vi "Transcriptor LabVIEW to VHDL code Step 0 Create Definitions.vi"(8 "error in":errorcluster, 11 "Diagram in":refnum<vi>) -> (0 "error out":errorcluster, 3 "structure definition cluster":T1)   [LabVIEW 2018]
uses:
  types/LabVIEW Universal Transcriptor Structure Definitions.ctl
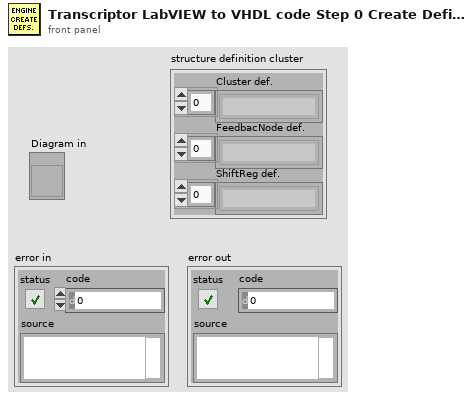
[diagram p1: front panel]
types:
  T1 = typedef "LabVIEW Universal Transcriptor Structure Definitions.ctl" = cluster{"Cluster def.":string[], "FeedbacNode def.":string[], "ShiftReg def.":string[]}
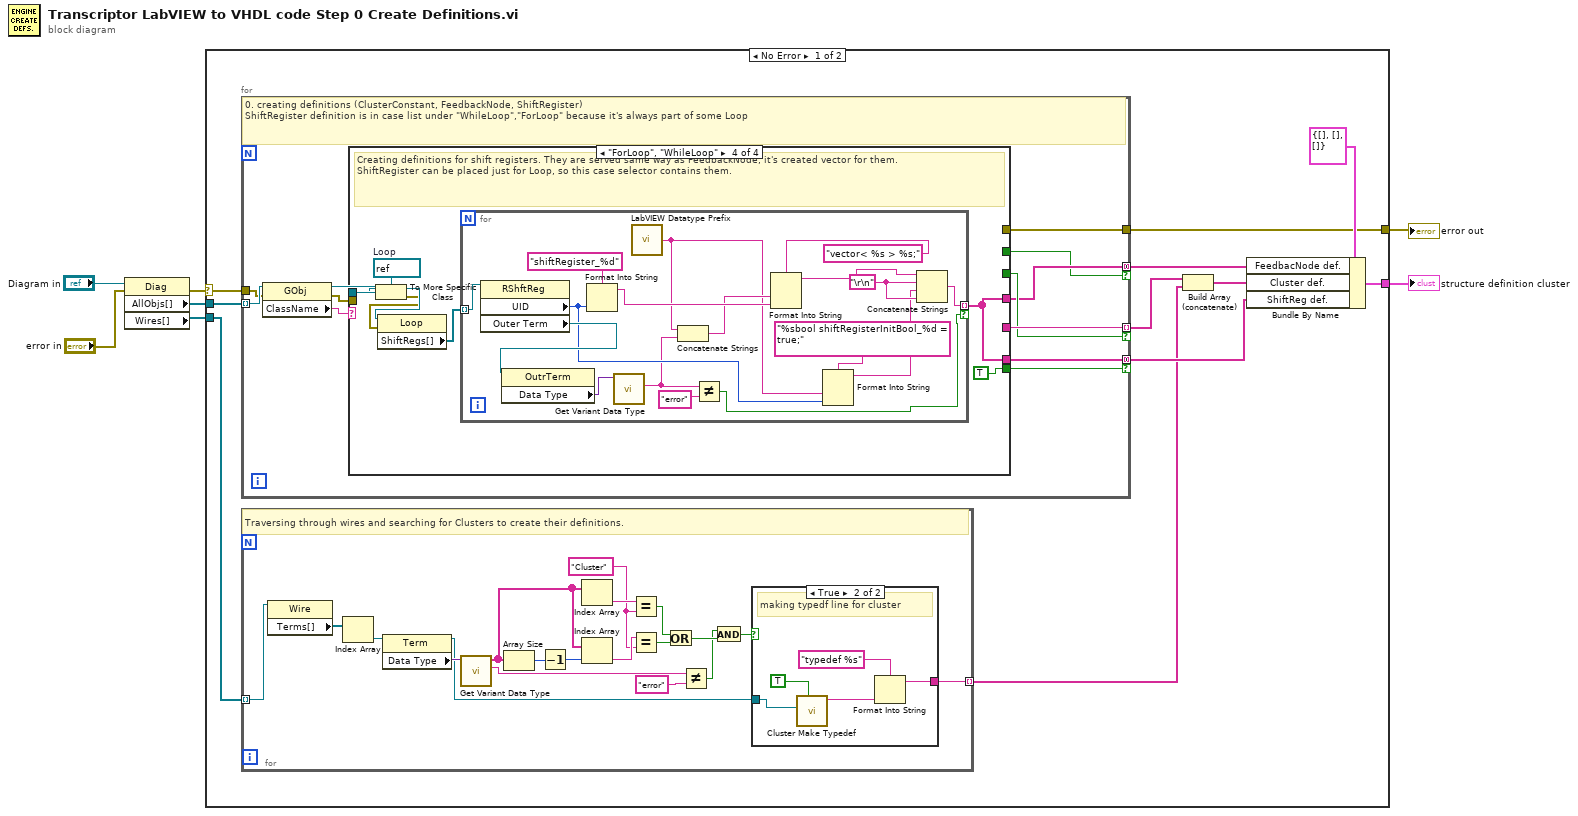
[diagram p0: block diagram]
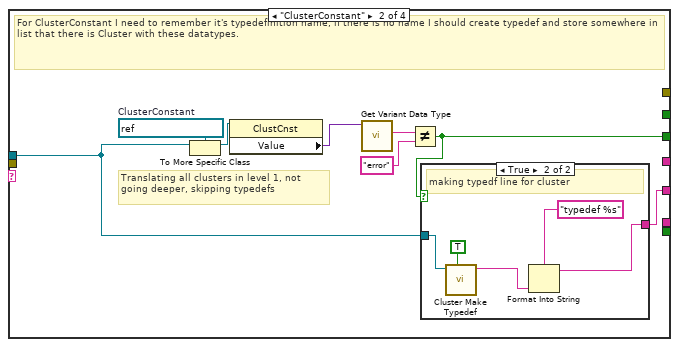
[diagram p4: hidden frame]
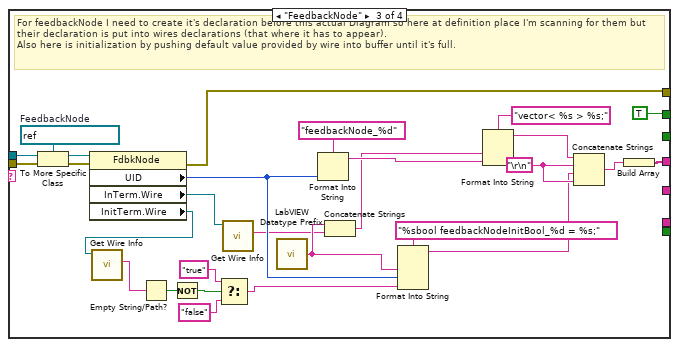
[diagram p6: hidden frame]
diagram:
  n1 = property class="Diag"(reference="Diagram in", error in="error in") -> (error out=w4:errorcluster, "AllObjs[]"=w7:refnum<vi>[], "Wires[]"=w1:refnum<vi>[])  [unwired: 1 out]
  n2 = case shown="No Error" w4 {
    selector: w4 -> [w14 w120]
    tunnel: [w18 _] -> w2
    tunnel: w7 -> [w15 _]
    tunnel: [w13 w120] -> w3
    tunnel: w1 -> [w11 _]
    frame No Error {
      n3 = for {
        tunnel: w15 -> [w54] mode=indexing
        tunnel: [w51] -> w10 mode=indexing if=w50
        tunnel: [w49] -> w17 mode=concatenating if=w48
        tunnel: w14 -> [w47]
        tunnel: [w45] -> w13
        tunnel: [w44] -> w12 mode=concatenating if=w43
        # "0. creating definitions (ClusterConstant, FeedbackNode, ShiftRegister)\nShiftRegister definition is in case list under \"WhileLoop\",\"ForLoop\" because it's always part of some Loop"
        n4 = property class="GObj"(reference=w54, error in=w47) -> (reference out=w52:refnum<vi>, error out=w46:errorcluster, "ClassName"=w53:string)
        n5 = case shown="\"ForLoop\", \"WhileLoop\"" w53 {
          tunnel: w52 -> [_ w57 w90 w99]
          tunnel: [_ w55 _ _] -> w51
          tunnel: [_ w58 _ _] -> w50
          tunnel: [_ _ w78 w97] -> w49
          tunnel: [_ _ TRUE _] -> w48
          tunnel: w46 -> [_ _ w69 _]
          tunnel: [_ _ w68 _] -> w45
          tunnel: [_ _ _ w97] -> w44
          tunnel: [_ _ _ TRUE] -> w43
          frame Default {
            # "If wire is not wired to anything from what I have to read value, output is default Variant value (hope that is empty Variant), and there will be just wire declaration without assignement in generated code."
          }
          frame "ClusterConstant" {
            w59 = refnum<vi> refnum  # ClusterConstant
            # "Translating all clusters in level 1, not going deeper, skipping typedefs"
            # "For ClusterConstant I need to remember it's typedefinition name, if there is no name I should create typedef and store somewhere in list that there is Cluster with these datatypes."
            n6 = To More Specific Class(target class=w59, reference=w57) -> (specific class reference=w56:refnum<vi>)  [unwired: 1 in, 1 out]
            n7 = property on="Property Node" class="ClustCnst"(reference=w56) -> ("Value"=w62:variant)  [unwired: 1 in, 2 out]
            n8 = call "Get Variant Data Type.vi"("Variant in"=w62) -> ("first data type"=w61:string)  [unwired: 9 in, 1 out]
            n9 = Not Equal?(x=w61, y="error") -> (x != y?=w58:bool)
            n10 = case shown="True" w58 {
              tunnel: w57 -> [_ w67]
              tunnel: [_ w64] -> w55
              frame False {
              }
              frame True {
                # "making typedf line for cluster"
                n11 = call "Cluster Make Typedef.vi"("skip first typedef?"=TRUE, "ClusterConstant refnum in"=w67) -> ("typedfinition"=w63:string)  [unwired: 7 in, 2 out]
                n12 = Format Into String(format string="typedef %s", w63) -> (resulting string=w64:string)  [unwired: 2 in, 1 out]
              }
            }
          }
          frame "FeedbackNode" {
            w84 = "\r\n"
            w95 = refnum<vi> refnum  # FeedbackNode
            # "For feedbackNode I need to create it's declaration before this actual Diagram so here at definition place I'm scanning for them but their declaration is put into wires declarations (that where it has to appear).\nAlso here is initialization by pushing default value provided by wire into buffer until it's full."
            n13 = To More Specific Class(target class=w95, reference=w90, error in=w69) -> (specific class reference=w94:refnum<vi>, error out=w93:errorcluster)
            n14 = property class="FdbkNode"(reference=w94, error in=w93) -> (error out=w68:errorcluster, "UID"=w85:i32, "InTerm.Wire"=w82:refnum<vi>, "InitTerm.Wire"=w71:refnum<vi>)  [unwired: 1 out]
            n15 = call "Get Wire Info.vi"("Wire"=w71) -> ("wire datatype"=w70:string)  [unwired: 9 in, 1 out]
            n16 = Empty String/Path?(string/path=w70) -> (empty?=w76:bool)
            n17 = Not(x=w76) -> (.not. x?=w75:bool)
            n18 = Select(t="true" ("format string"), s=w75, f="false" ("format string")) -> (s? t:f=w72:string)
            n19 = call "Get Wire Info.vi"("Wire"=w82) -> ("wire datatype"=w77:string)  [unwired: 9 in, 1 out]
            n20 = call "LabVIEW Datatype Prefix.vi"() -> ("datatype prefix"=w80:string)
            n21 = Format Into String(format string="feedbackNode_%d", w85) -> (resulting string=w87:string)  [unwired: 2 in, 1 out]
            n22 = Concatenate Strings(w80, w77) -> (w81:string)
            n23 = Format Into String(format string="%sbool feedbackNodeInitBool_%d = %s;", w80, w85, w72) -> (resulting string=w83:string)  [unwired: 2 in, 1 out]
            n24 = Format Into String(format string="vector< %s > %s;", w81, w87) -> (resulting string=w88:string)  [unwired: 2 in, 1 out]
            n25 = Concatenate Strings(w88, w84, w83, w84) -> (w79:string)
            n26 = Build Array(w79) -> (w78:string[])
          }
          frame "ForLoop", "WhileLoop" {
            w102 = refnum<vi> refnum  # Loop
            # "Creating definitions for shift registers. They are served same way as FeedbackNode, it's created vector for them.\nShiftRegister can be placed just for Loop, so this case selector contains them."
            n27 = To More Specific Class(target class=w102, reference=w99) -> (specific class reference=w101:refnum<vi>, error out=w100:errorcluster)  [unwired: 1 in]
            n28 = property class="Loop"(reference=w101, error in=w100) -> ("ShiftRegs[]"=w98:refnum<vi>[])  [unwired: 2 out]
            n29 = for {
              tunnel: w98 -> [w119] mode=indexing
              tunnel: [w108] -> w97 mode=indexing if=w105
              w111 = "\r\n"
              n30 = property class="RShftReg"(reference=w119) -> ("UID"=w107:i32, "Outer Term"=w116:refnum<vi>)  [unwired: 1 in, 2 out]
              n31 = property class="OutrTerm"(reference=w116) -> ("Data Type"=w104:variant)  [unwired: 1 in, 2 out]
              n32 = Format Into String(format string="shiftRegister_%d", w107) -> (resulting string=w117:string)  [unwired: 2 in, 1 out]
              n33 = call "Get Variant Data Type.vi"("Variant in"=w104) -> ("first data type"=w103:string)  [unwired: 9 in, 1 out]
              n34 = call "LabVIEW Datatype Prefix.vi"() -> ("datatype prefix"=w112:string)
              n35 = Concatenate Strings(w112, w103) -> (w114:string)
              n36 = Not Equal?(x=w103, y="error") -> (x != y?=w105:bool)
              n37 = Format Into String(format string="vector< %s > %s;", w114, w117) -> (resulting string=w110:string)  [unwired: 2 in, 1 out]
              n38 = Format Into String(format string="%sbool shiftRegisterInitBool_%d = true;", w112, w107) -> (resulting string=w109:string)  [unwired: 2 in, 1 out]
              n39 = Concatenate Strings(w110, w111, w109, w111) -> (w108:string)
            }
          }
        }
      }
      n40 = for {
        tunnel: w11 -> [w21] mode=indexing
        tunnel: [w20] -> w9 mode=indexing
        w26 = "Cluster" ("y")
        # "Traversing through wires and searching for Clusters to create their definitions."
        n41 = property on="Property Node" class="Wire"(reference=w21) -> ("Terms[]"=w35:refnum<vi>[])  [unwired: 1 in, 2 out]
        n42 = Index Array(array=w35) -> (element=w34:refnum<vi>)  [unwired: 1 in]
        n43 = property on="Property Node" class="Term"(reference=w34) -> (reference out=w19:refnum<vi>, "Data Type"=w33:variant)  [unwired: 1 in, 1 out]
        n44 = call "Get Variant Data Type.vi"("Variant in"=w33) -> ("first data type"=w37:string, "Data Types[]"=w30:string[])  [unwired: 9 in]
        n45 = Array Size(array=w30) -> (size(s)=w32:i32)
        n46 = Decrement(x=w32) -> (x-1=w31:i32)
        n47 = Index Array(array=w30) -> (element=w28:string)  [unwired: 1 in]
        n48 = Index Array(array=w30, index=w31) -> (element=w27:string)
        n49 = Equal?(x=w28, y=w26) -> (x = y?=w25:bool)
        n50 = Equal?(x=w27, y=w26) -> (x = y?=w29:bool)
        n51 = Or(x=w25, y=w29) -> (x .or. y?=w24:bool)
        n52 = Not Equal?(x=w37, y="error") -> (x != y?=w23:bool)
        n53 = And(x=w23, y=w24) -> (x .and. y?=w22:bool)
        n54 = case shown="True" w22 {
          tunnel: w19 -> [_ w38]
          tunnel: [_ w40] -> w20
          frame False {
          }
          frame True {
            # "making typedf line for cluster"
            n55 = call "Cluster Make Typedef.vi"("skip first typedef?"=TRUE, "Terminal in"=w38) -> ("typedfinition"=w39:string)  [unwired: 7 in, 2 out]
            n56 = Format Into String(format string="typedef %s", w39) -> (resulting string=w40:string)  [unwired: 2 in, 1 out]
          }
        }
      }
      n57 = Build Array (concatenate)(w10, w9) -> (w8:string[])
      n58 = Bundle By Name(cluster=T1 {"Cluster def."=[], "FeedbacNode def."=[], "ShiftReg def."=[]} ("Defines Cluster"), "FeedbacNode def."=w17, "Cluster def."=w8, "ShiftReg def."=w12) -> (w18:T1)
    }
    frame Error {
    }
  }
  "error out" <- w3
  "structure definition cluster" <- w2
